vi "Decode.vi"(8 "error in (no error)":errorcluster, 10 "Binary string in":string, 11 "obj in":refnum<class "FrameInfo.lvclass">) -> (0 "error out":errorcluster, 1 "Data out":refnum<class "Data.lvclass">, 2 "Rest of binary string":string, 3 "obj out":refnum<class "FrameInfo.lvclass">)   [LabVIEW 2020, in "FrameInfo.lvclass"]
uses:
  FrameInfo.lvclass
  Data Class/Data.lvclass
  Data Class/Datatypes/Data_FrameInfo_class/Attribute.vi
  FrameInfo.lvclass/FrameInfo.ctl
  Data Class/Datatypes/Data_FrameInfo_class/Data_FrameInfo.lvclass
  C:/Users/theod/Desktop/API - EyeT data streaming to IC/Smart Eye API/Source/Classes/Smart Eye Pro Drivers/Data Class/Data.lvclass
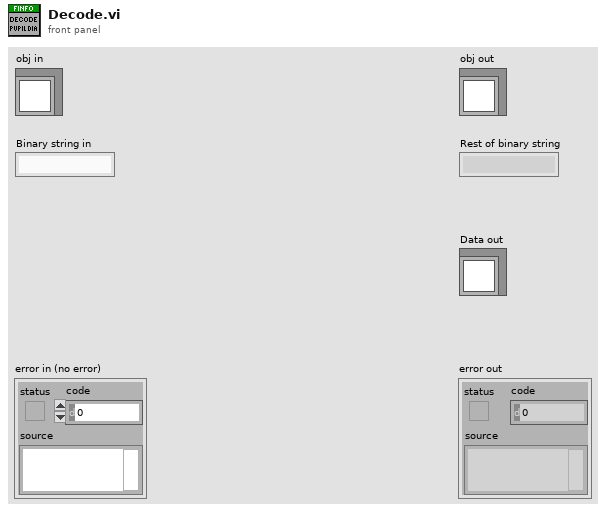
[diagram p1: front panel]
types:
  T1 = typedef "Data_FrameInfo.lvclass/Attribute.vi" = cluster{"TimeStamp":u64}
  T2 = enum16{"big-endian, network order", "native, host order", "little-endian"}
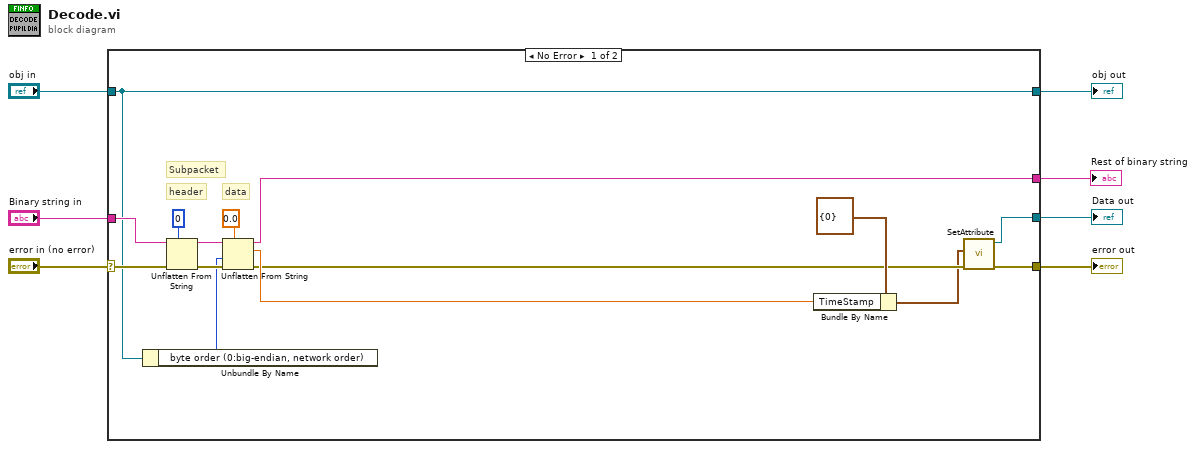
[diagram p0: block diagram]
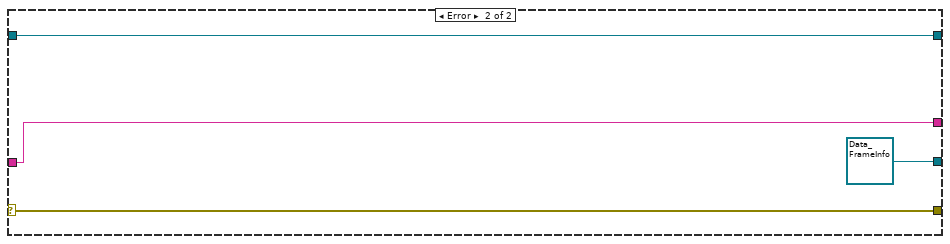
[diagram p2: hidden frame]
diagram:
  n1 = case shown="No Error" "error in (no error)" {
    selector: "error in (no error)" -> [w18 w26]
    tunnel: [w13 w26] -> w6
    tunnel: "obj in" -> [w9 w25]
    tunnel: [w9 w25] -> w4
    tunnel: "Binary string in" -> [w16 w23]
    tunnel: [w11 refnum<class "Data_FrameInfo.lvclass"> refnum ("Data_General out")] -> w2
    tunnel: [w10 w23] -> w1
    frame No Error {
      # "header"
      # "data"
      # "Subpacket"
      n2 = Unbundle By Name(w9) -> ("byte order (0:big-endian, network order)"=w8:T2)
      n3 = Unflatten From String(type=u32 0, binary string=w16, error in (no error)=w18) -> (rest of the binary string=w22:string, error out=w19:errorcluster)  [unwired: 2 in, 1 out]
      n4 = Unflatten From String(type=0.0, binary string=w22, byte order (0:big-endian, network order)=w8, error in (no error)=w19) -> (rest of the binary string=w10:string, value=w17:dbl, error out=w14:errorcluster)  [unwired: 1 in]
      n5 = Bundle By Name(cluster=T1 {"TimeStamp"=0} ("Attribute"), "TimeStamp"=w17) -> (w12:T1)
      n6 = call "SetAttribute.vi"("error in (no error)"=w14, "Set Attribute"=w12) -> ("error out"=w13:errorcluster, "Data_General out"=w11:refnum<class "Data_FrameInfo.lvclass">)  [unwired: 8 in]
    }
    frame Error {
    }
  }
  "error out" <- w6
  "obj out" <- w4
  "Data out" <- w2
  "Rest of binary string" <- w1
